vi "Get Spool Progress.vi"(8 "error in (no error)":errorcluster, 11 "index":i32) -> (0 "error out":errorcluster, 2 "function return":u32, 3 "index out":i32)   [LabVIEW 2014, in "atmcd32d.lvlib"]
doc: "unsigned int WINAPI GetSpoolProgress(long * index);"
uses:
  atmcd32d.lvlib
  atmcd32d.dll
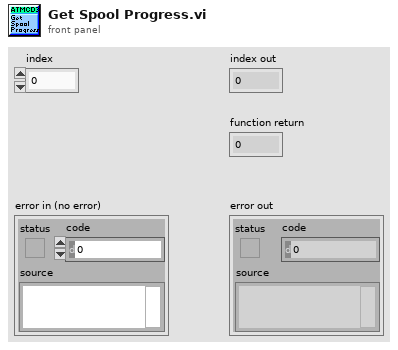
[diagram p1: front panel]
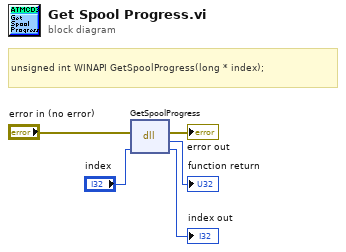
[diagram p0: block diagram]
diagram:
  # "unsigned int WINAPI GetSpoolProgress(long * index);"
  n1 = dll-call lib="C:/Users/Bakir/Documents/Lambda2-Testing/lib/Andorlib/atmcd32d.*" fn="GetSpoolProgress"(error in="error in (no error)", "index"="index") -> (error out=→"error out":errorcluster, →"function return":u32, "index"=→"index out":i32)  [unwired: 2 in, 1 out]
